vi "Navigation_no s curve may 2 encoders with mining.vi"() -> ()   [LabVIEW 2015]
uses:
  <vilib>/myRIO/Instrument Drivers/Onboard IO/PWM/typedefs/PWM Reference.ctl
  <vilib>/myRIO/Common/Instrument Driver Framework/Utilities/typedefs/myRIO Generic Hardware Reference.ctl
  <vilib>/myRIO/Common/Instrument Driver Framework/Utilities/typedefs/Hardware Version Enum.ctl
  <vilib>/myRIO/Common/Instrument Driver Framework/Utilities/typedefs/myRIO v1.0 Reference.ctl
  <vilib>/myRIO/Common/Instrument Driver Framework/Utilities/typedefs/Generic FPGA Reference.ctl
  <vilib>/myRIO/Common/Instrument Driver Framework/myRIO v1.0/PWM/typedefs/PWM Channels Enum.ctl
  <vilib>/myRIO/Instrument Drivers/Onboard IO/PWM/typedefs/PWM Configuration.ctl
  <vilib>/userdefined/High Color/nirio_resource_hc.ctl
  <vilib>/myRIO/Common/Instrument Driver Framework/myRIO v1.0/PWM/vis/myRIO v1.1 Open PWM.vi
  <vilib>/myRIO/Common/Instrument Driver Framework/Utilities/vis/Validate Channels.vi
  <vilib>/myRIO/Common/Instrument Driver Framework/myRIO v1.0/PWM/vis/myRIO v1.0 Reserve PWM.vi
  <vilib>/myRIO/Common/Instrument Driver Framework/myRIO v1.0/PWM/vis/myRIO v1.0 Build MUX Configuration PWM.vi
  <vilib>/myRIO/Common/Instrument Driver Framework/myRIO v1.0/Resource Manager/vis/myRIO v1.0 Reserve Channel List.vi
  <vilib>/myRIO/Common/Instrument Driver Framework/myRIO v1.0/Resource Manager/vis/myRIO v1.0 Create Configuration List.vi
  <vilib>/myRIO/Common/Instrument Driver Framework/myRIO v1.0/Resource Manager/vis/myRIO v1.0 Reserve Channel.vi
  <vilib>/myRIO/Common/Instrument Driver Framework/myRIO v1.0/Resource Manager/vis/myRIO v1.0 Unreserve Channel.vi
  <vilib>/myRIO/Common/Instrument Driver Framework/myRIO v1.0/Resource Manager/vis/myRIO v1.0 Build Mutex Name.vi
  <vilib>/FPGAPlugInAG/myRIO-1900/niLvFpga_Open_myRIO-1900.vi
  <vilib>/rvi/interface/common/dynamic/niFpgaDynamicAddResources.vi
  <vilib>/myRIO/Common/Instrument Driver Framework/Utilities/vis/FPGA Ref Manager.vi
  <vilib>/Utility/error.llb/Error Cluster From Error Code.vi
  <vilib>/myRIO/Common/Instrument Driver Framework/Utilities/vis/Ref Counter.vi
  <vilib>/rvi/errors/niLvFpgaAdjustHostInterfaceError.vi
  <vilib>/Utility/VariantDataType/GetNumericInfo.vi
  <vilib>/myRIO/Common/Instrument Driver Framework/myRIO v1.0/myRIO v1.1 Open.vi
  <vilib>/myRIO/Common/Instrument Driver Framework/Utilities/vis/IO Manager.vi
  <vilib>/myRIO/Common/Instrument Driver Framework/Utilities/vis/Configuration Manager.vi
  <vilib>/myRIO/Common/Instrument Driver Framework/myRIO v1.0/Resource Manager/vis/myRIO v1.0 Configure IO.vi
  <vilib>/myRIO/Common/Instrument Driver Framework/myRIO v1.0/myRIO v1.0 Close.vi
  <vilib>/myRIO/Common/Instrument Driver Framework/myRIO v1.0/PWM/vis/myRIO v1.0 Write PWM.vi
  <vilib>/addons/control/pid/pid.llb/PID (DBL).vi
  <vilib>/rvi/interface/nirviOpenFPGA/nirviOpenFPGA.xnode
  FPGA Bitfiles/NavigationProjec_FPGATarget2_FPGAMainNavigati_PWPHW8gwDxI.lvbitx
  <vilib>/rvi/interface/nirviReadWriteControl/nirviReadWriteControl.xnode
  <vilib>/myRIO/Instrument Drivers/Onboard IO/PWM/vis/myRIO PWM Open.xnode
  <vilib>/myRIO/Instrument Drivers/Onboard IO/PWM/PWM.lvlib
  <vilib>/myRIO/Instrument Drivers/Utilities/Utilities.lvlib
  NiFpgaLv.dll
  <vilib>/rvi/interface/Simulation/niFpgaSimulationCallBeginRW.vi
  <vilib>/addons/control/pid/NI_PID_pid.lvlib
panel:
  in  "Tab Control":enum32{"Page 1", "Page 2"}(tab)
  out "percent to goal":dbl
  out "x goal current":dbl=8.0
  out "big red button":i16
  out "y1ahead":dbl
  out "angle error":dbl
  out "y desired":dbl
  out "slope desired":dbl
  out "orientation theta desired":dbl
  out "current angle":dbl
  out "current y":dbl
  out "current x":dbl
  out "mining angle":dbl
  out "mining y":dbl
  out "mining x":dbl
  out "mining location":dbl=1.0
  out "distance to goal":dbl
  out "loc_y":dbl
  out "loc_x":dbl
  out "loc_theta":dbl
  in  "motor killswitch":bool=TRUE
  in  "set start position":bool
  in  "dumping complete":bool
  in  "digging complete?":bool
  in  "position good?":bool
  in  "state":dbl
  in  "x goal":dbl=8.0
  in  "Encoder Reset":bool
  out "scale":dbl=1.0
  out "reset x y 2":dbl
  out "stop motors":dbl
  out "encoder stop switch":dbl=1.0
  out "left wheels actual pwm":dbl
  out "right wheels actual pwm":dbl
  out "desired pwm right":dbl
  out "desired pwm left":dbl
  out "left setpoint":dbl
  out "right setpoint":dbl
  in  "PID Settings":enum32{"Right PID PWM", "Left PID PWM"}(tab)
  in  "output range right":cluster{"output high":dbl, "output low":dbl}={"output high"=0.13333, "output low"=-0.13333} {"output low" format="%.6f"; "output high" format="%.5f"}
  in  "PID gains right":T1={"proportional gain (Kc)"=0.002, "integral time (Ti, min)"=7e-07, "derivative time (Td, min)"=0.0} {"derivative time (Td, min)" format="%.8f"; "integral time (Ti, min)" format="%.8f"; "proportional gain (Kc)" format="%.8f"}
  out "dt out (s) right":dbl format="%.3f"
  out "PID feedback Right":dbl
  out "Elapsed Time (s) Right":dbl caption="Elapsed Time (s)"
  in  "pid reset right":bool
  in  "output range left":cluster{"output high":dbl, "output low":dbl}={"output high"=0.13333, "output low"=-0.13333} {"output low" format="%.6f"; "output high" format="%.5f"}
  in  "PID gains left":T1={"proportional gain (Kc)"=0.002, "integral time (Ti, min)"=7e-07, "derivative time (Td, min)"=0.0} {"derivative time (Td, min)" format="%.8f"; "integral time (Ti, min)" format="%.8f"; "proportional gain (Kc)" format="%.8f"}
  out "dt out (s) left":dbl format="%.3f"
  out "PID feedback Left":dbl
  out "Elapsed Time (s) Left":dbl caption="Elapsed Time (s)"
  in  "pid reset left":bool
  out "start angle":dbl=1.0
  out "start x":dbl=1.0
  out "start y":dbl
  in  "stuff that i dont want to mess with right now":T2(tab)
  out "RM Linear Velocity (rot/s)":dbl
  out "RR Rot Velocity (rot/s)":dbl
  out "LR Rot Velocity (rot/s)":dbl
  out "LM Rot Velocity (rot/s)":dbl
  out "LF Rot Velocity (rot/s)":dbl
  out "RF Linear Velocity (rot/s)":dbl
  out "Tick Count(mSec) 2":u32 caption="Tick Count(mSec)"
  out "y traveled 2":dbl
  out "x traveled 2":dbl
  out "y position 2":dbl
  out "x position 2":dbl
  out "y dot 2":dbl
  out "distance traveled 2":dbl
  out "psi dot 2":dbl
  out "x dot 2":dbl
  out ".not. x? 2":bool
  out ".not. x? 3":bool
  out "goal reached":bool=TRUE
  out "avg ENC.B":dbl
  out "avg ENC.A":dbl
  out "ENC.B_c.CNTR":i32
  out "ENC.B_b.CNTR":i32
  out "ENC.B_a.CNTR":i32
  out "ENC.A_c.CNTR":i32
  out "ENC.A_b.CNTR":i32
  out "ENC.A_a.CNTR":i32
  out "stage set point parameters":T3(tab)
  in  "x straight 1 end":dbl=2.0
  in  "ypstart straight 1":dbl
  in  "ystart":dbl=1.0
  in  "yend straight 1":dbl=2.0
  in  "ypend straight 1":dbl
  out "a":dbl
  out "b":dbl
  out "c":dbl
  out "d":dbl
  out "x turn end":dbl=7.0
  out "x straight 2 end":dbl=10.0
  in  "mining y 1":dbl=2.0
  in  "mining angle 1":dbl
  in  "mining x 1":dbl=-8.0
  in  "mining angle -1":dbl
  in  "mining y -1":dbl=4.0
  in  "mining x -1":dbl=-8.0
  out "left pwm":dbl(graph)
  out "right pwm":dbl(graph)
  out "SYS.SELECTA":u8 format="%08b"
  in  "R Min Linear Velocity (ft/s)":dbl=-2.0 format="%#_13g"
  in  "R Max Linear Velocity (ft/s)":dbl=2.0 format="%#_13g"
  in  "L Min Linear Velocity (ft/s)":dbl=-2.0 format="%#_13g"
  in  "L Max Linear Velocity (ft/s)":dbl=2.0 format="%#_13g"
  out "Current Rot Velocity (rot/s)":T4(graph)
  # "Position Information"
  # "move cases along"
  # "end state 0\ngo to state 1"
  # "end state 1\ngo to state 2"
  # "end state 2\ngo to state 3"
  # "end state 3\ngo to state 4"
  # "end state 4\ngo to state 0"
  # "same thing, redundant \nbut can be changed to \nsomething useful later"
  # "this must be true to \ninitialize the routine"
  # "go through the 3\n movement cases"
  # "go through the 3\n movement cases"
  # "Stop Flags \n1=go \n0=stop"
  # "PWM Setpoint"
  # "Initial condtions"
  # "Encoder Values"
  # "Motor Control Parameters"
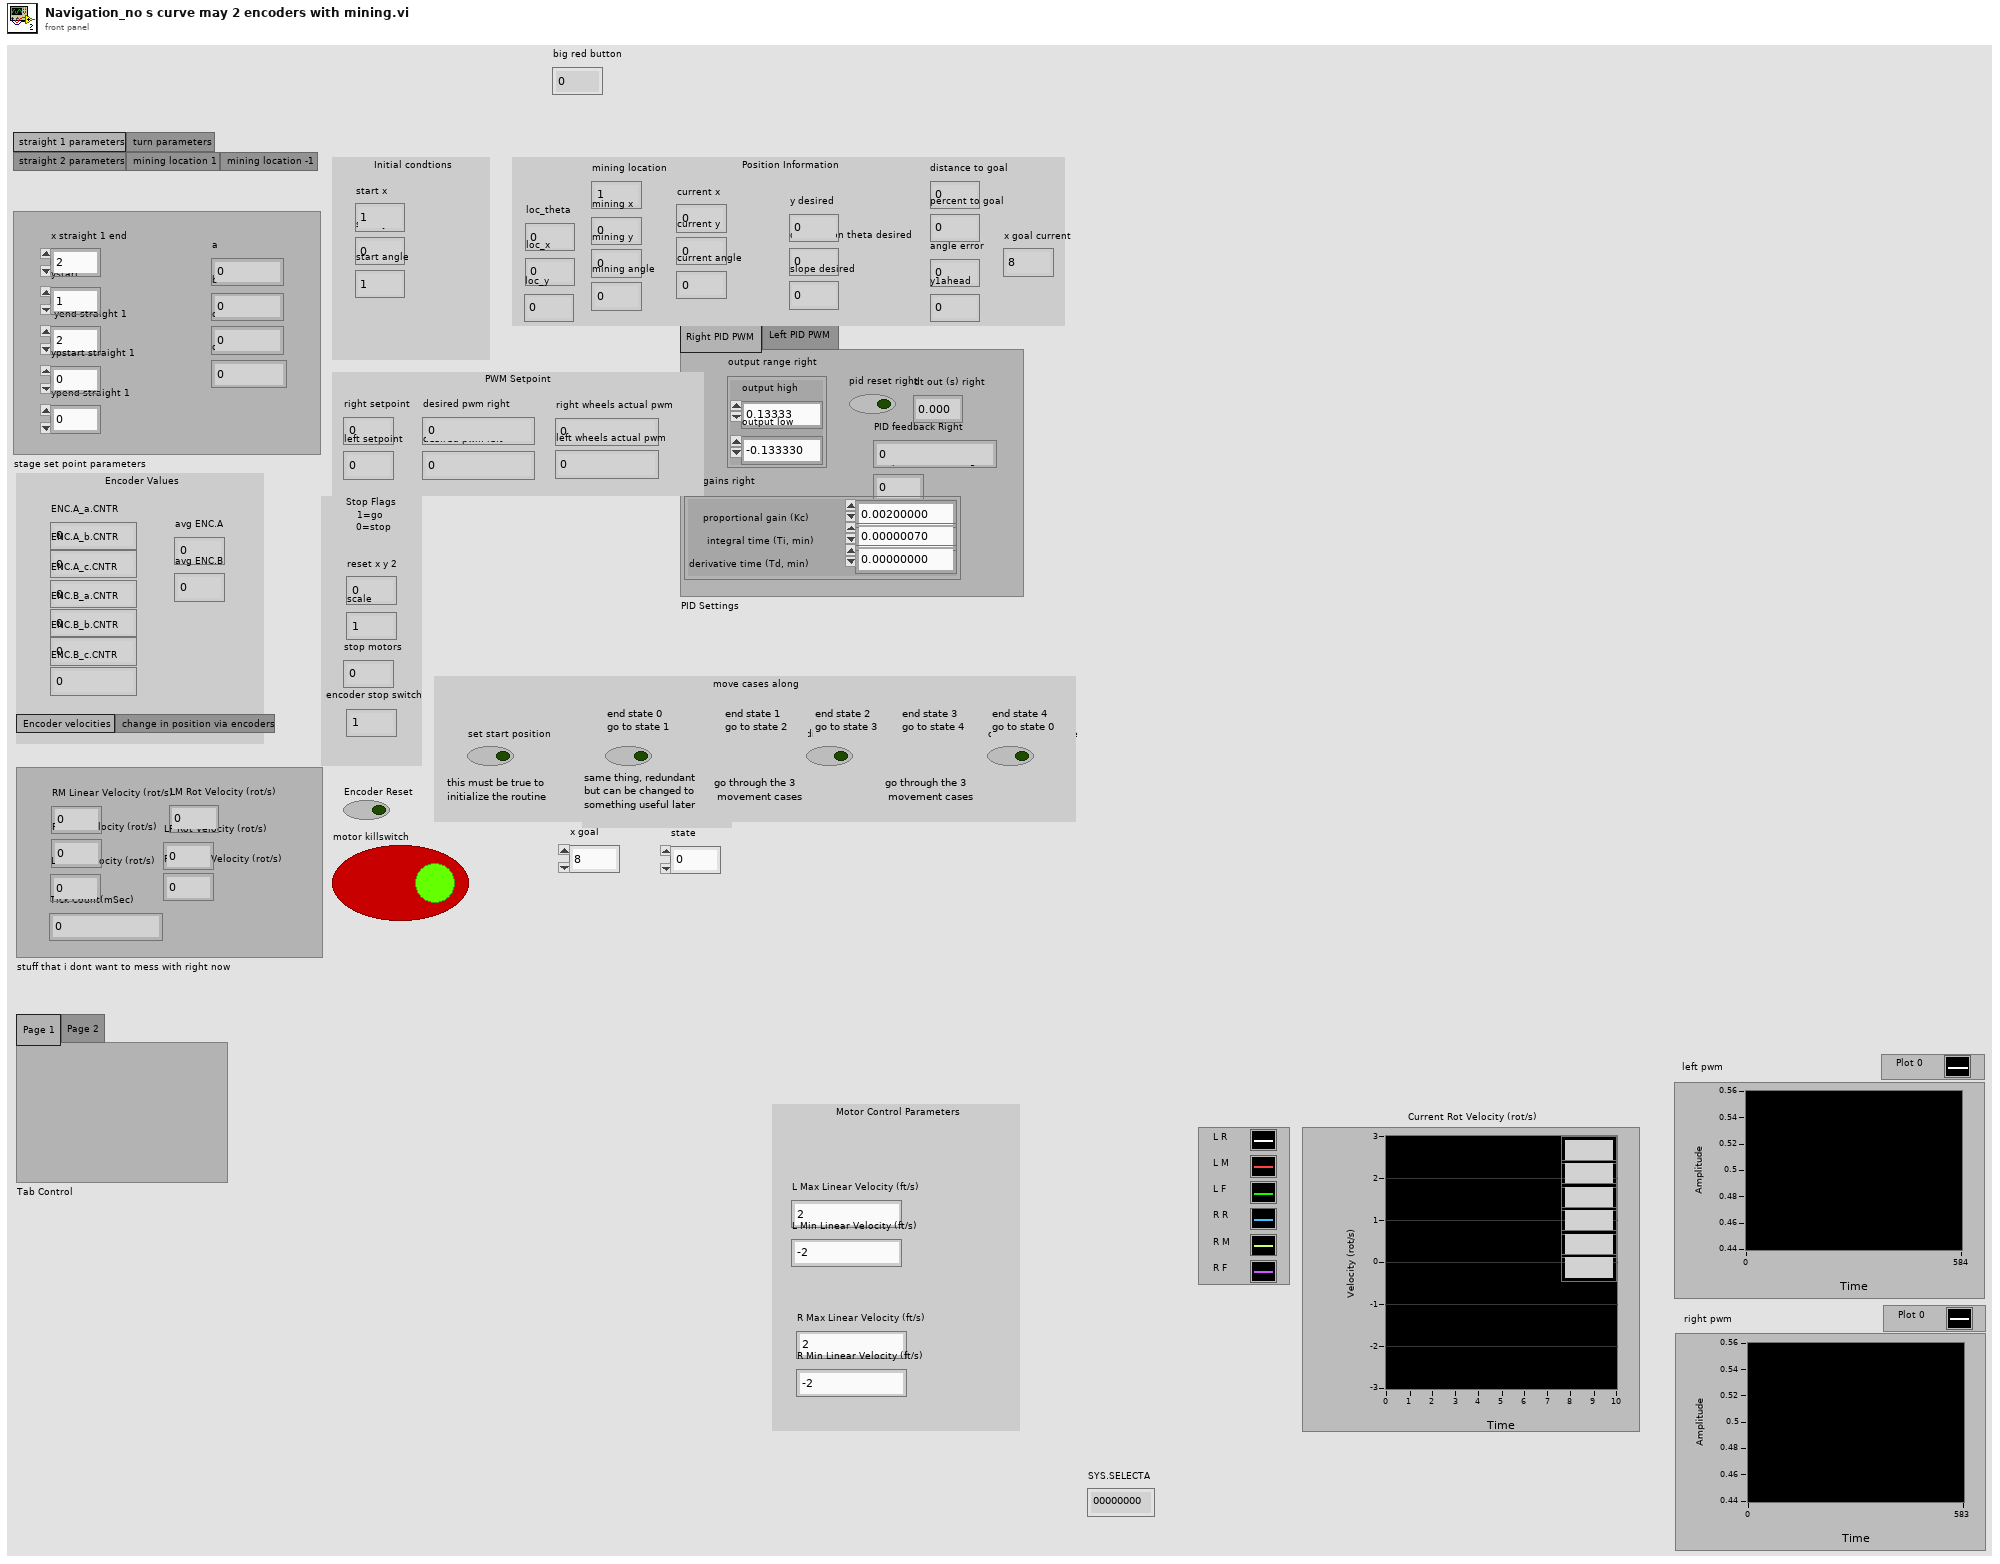
[diagram p1: front panel]
types:
  T1 = cluster{"proportional gain (Kc)":dbl, "integral time (Ti, min)":dbl, "derivative time (Td, min)":dbl}
  T2 = enum32{"Encoder velocities", "change in position via encoders"}
  T3 = enum32{"straight 1 parameters", "turn parameters", "straight 2 parameters", "mining location 1", "mining location -1"}
  T4 = cluster{"Rotational Velocity (RPS)":dbl, "Rotational Velocity (RPS)":dbl, "Rotational Velocity (RPS)":dbl, "Rotational Velocity (RPS)":dbl, "Rotational Velocity (RPS)":dbl, "Rotational Velocity (RPS)":dbl}
  T5 = typedef "nirio_resource_hc.ctl" = tag
  T6 = typedef "Hardware Version Enum.ctl" = enum16{"Unknown", "myRIO-1900", "myRIO-1950", "roboRIO"}
  T7 = typedef "PWM.lvlib/PWM Reference.ctl" = cluster{"myRIO Reference":T8, "PWM Channels Enum":T11, "PWM Configuration":T12}
  T8 = typedef "myRIO Generic Hardware Reference.ctl" = cluster{"myRIO Model":T6, "myRIO Hardware Reference":T9}
  T9 = typedef "myRIO v1.0 Reference.ctl" = cluster{"Generic FPGA Reference":T10, "Allow multiple opens":bool}
  T10 = typedef "Generic FPGA Reference.ctl" = refnum<k20>
  T11 = typedef "PWM Channels Enum.ctl" = enum16{"Not Connected", "C/PWM0", "C/PWM1", "A/PWM0", "A/PWM1", "A/PWM2", "B/PWM0", "B/PWM1", "B/PWM2", "PWM/PWM0", "PWM/PWM1", "PWM/PWM2", "PWM/PWM3", "PWM/PWM4", "PWM/PWM5", "PWM/PWM6", "PWM/PWM7", "PWM/PWM8", "PWM/PWM9"}
  T12 = typedef "PWM.lvlib/PWM Configuration.ctl" = cluster{"Frequency":dbl, "Duty Cycle":dbl}
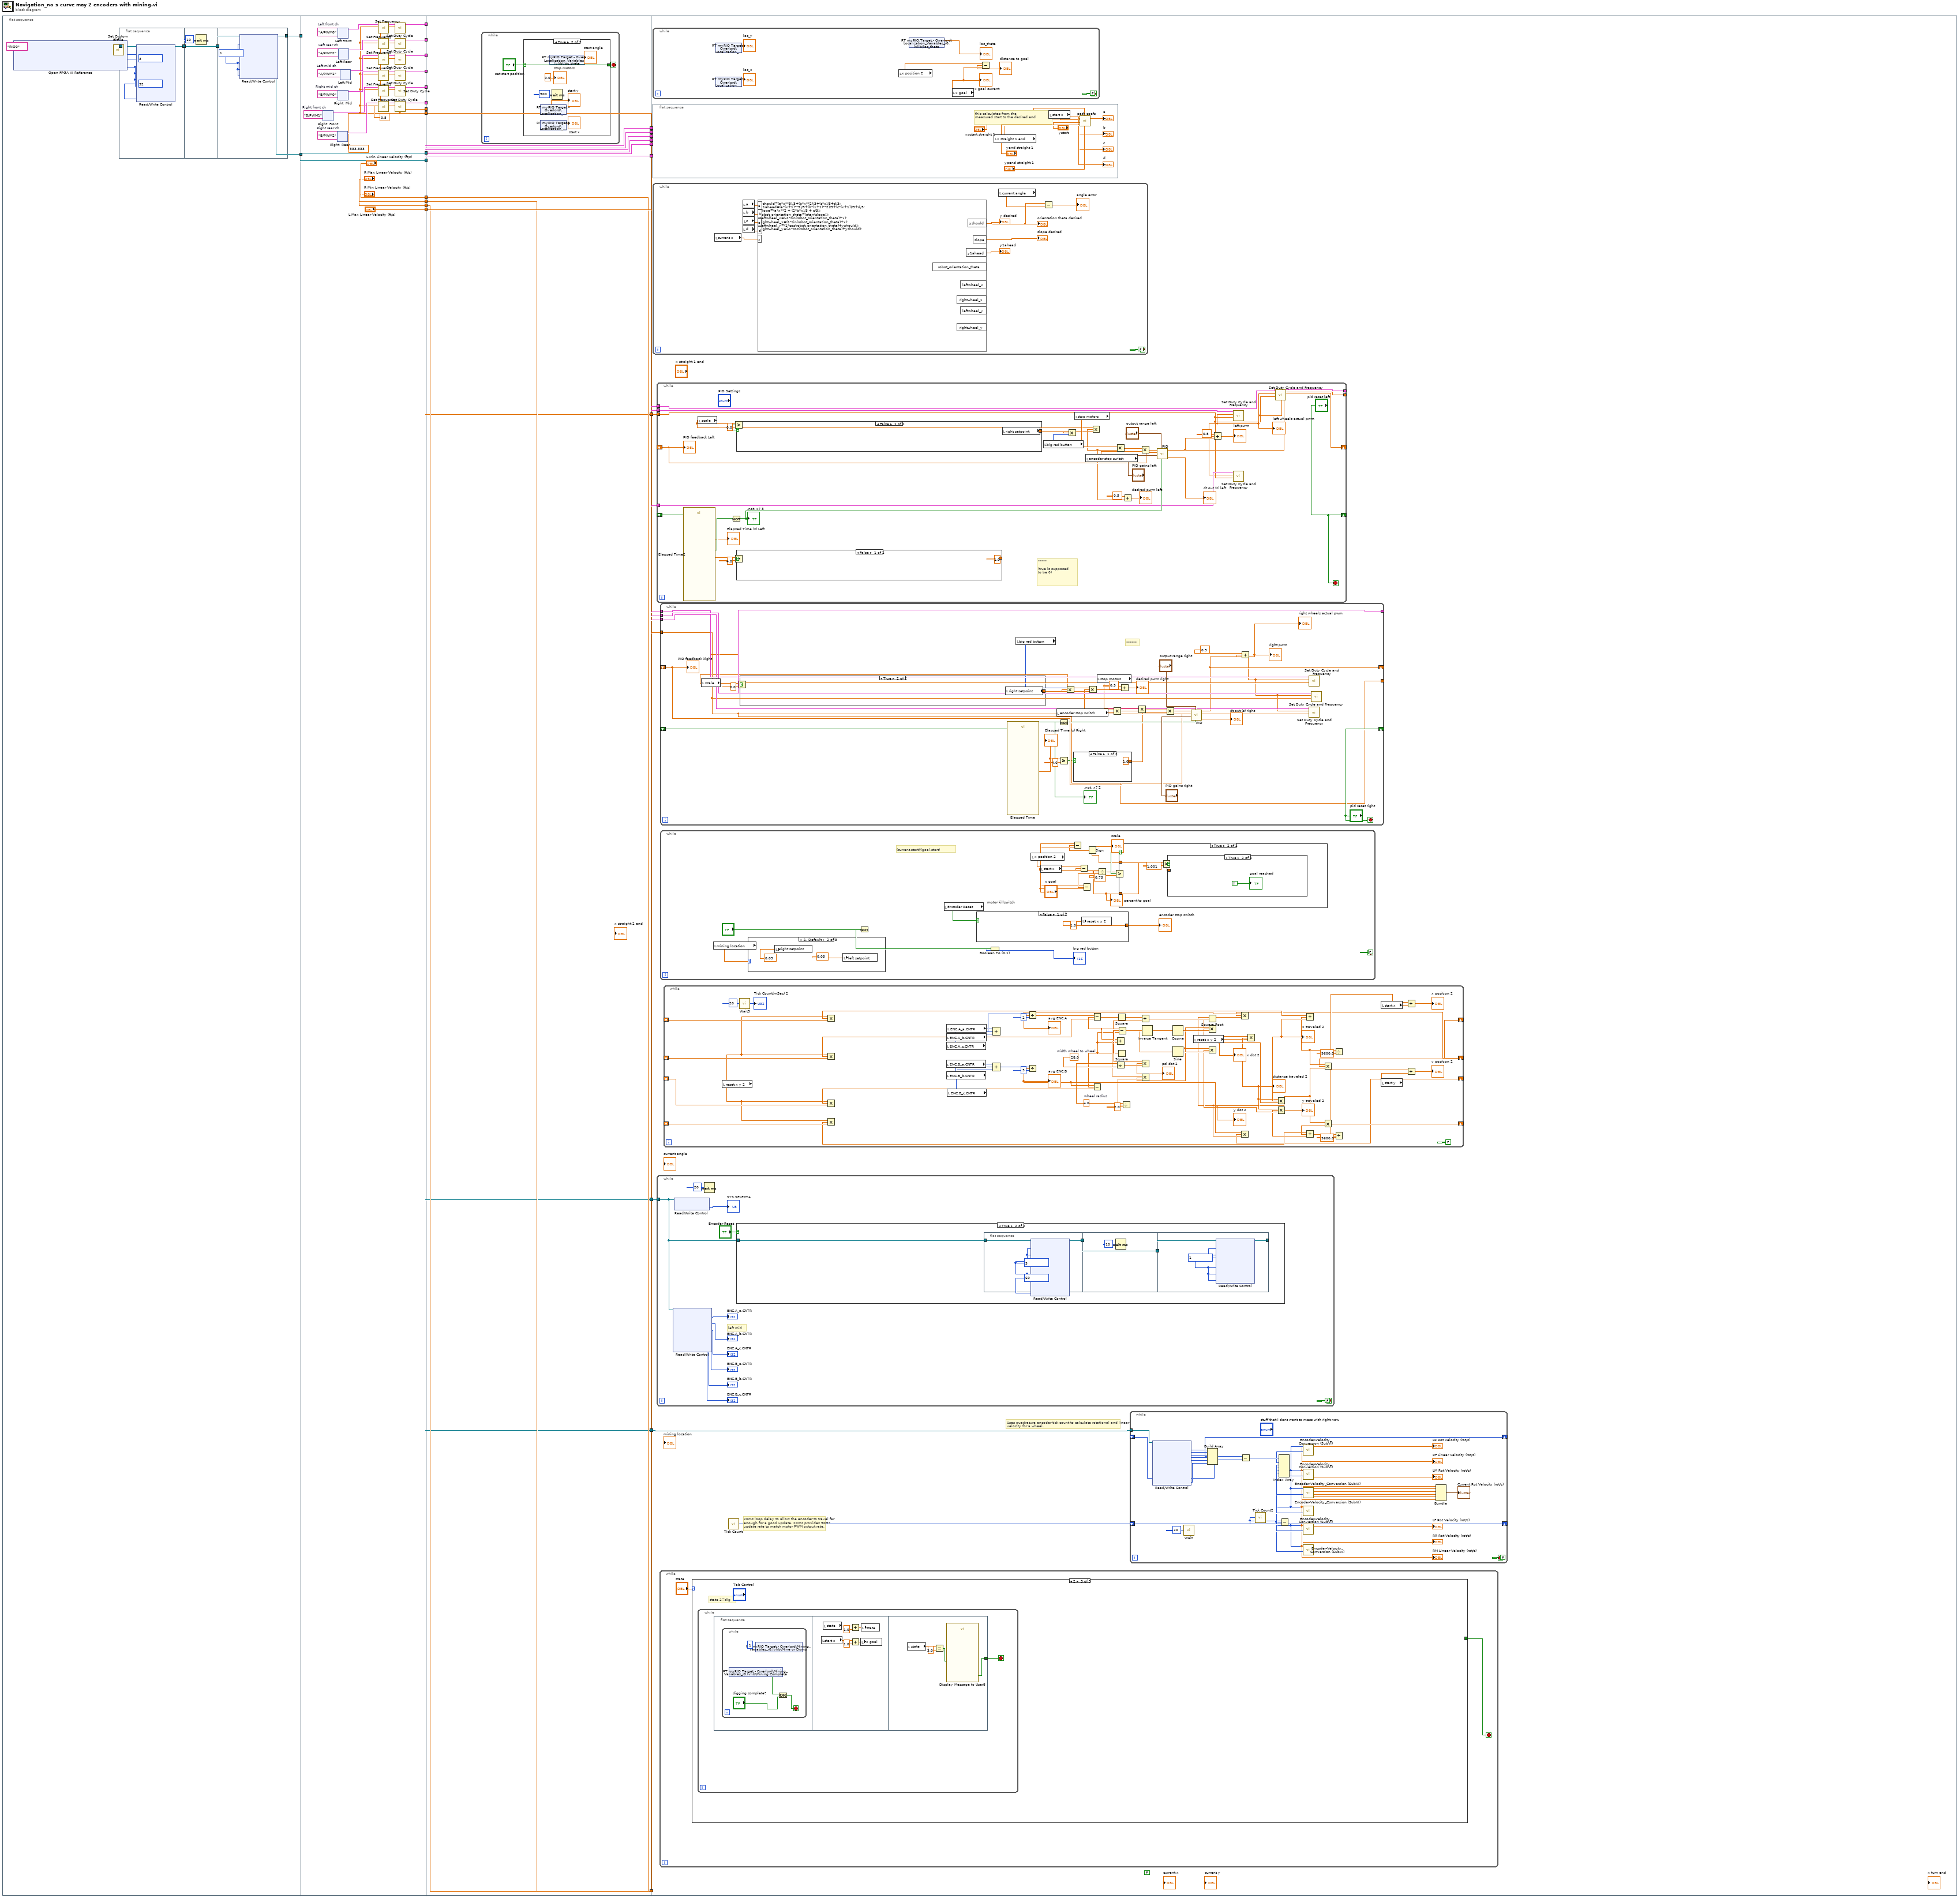
[diagram p0: block diagram]
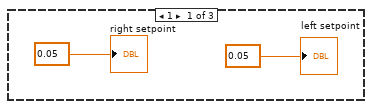
[diagram p3: hidden frame]
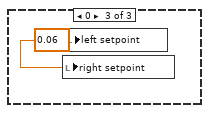
[diagram p4: hidden frame]
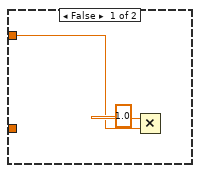
[diagram p5: hidden frame]
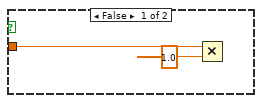
[diagram p6: hidden frame]
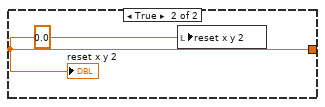
[diagram p7: hidden frame]
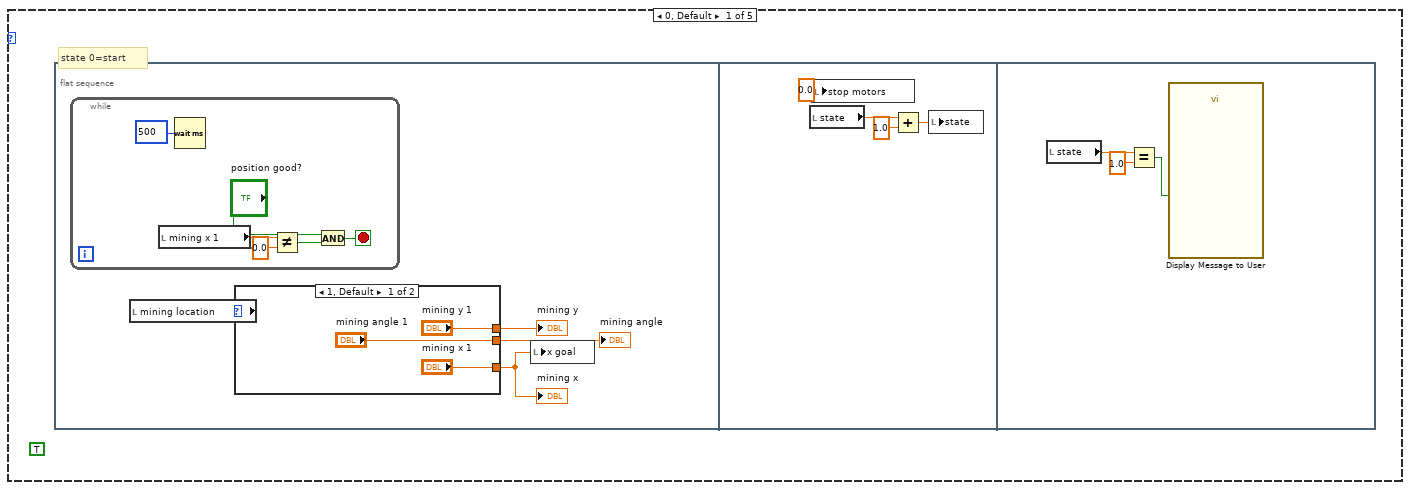
[diagram p8: hidden frame]
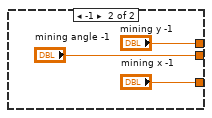
[diagram p9: hidden frame]
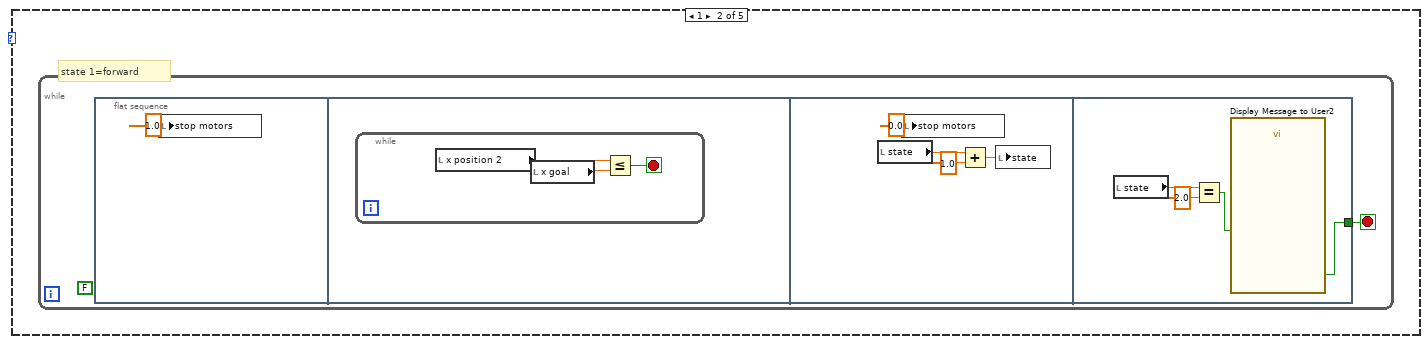
[diagram p10: hidden frame]
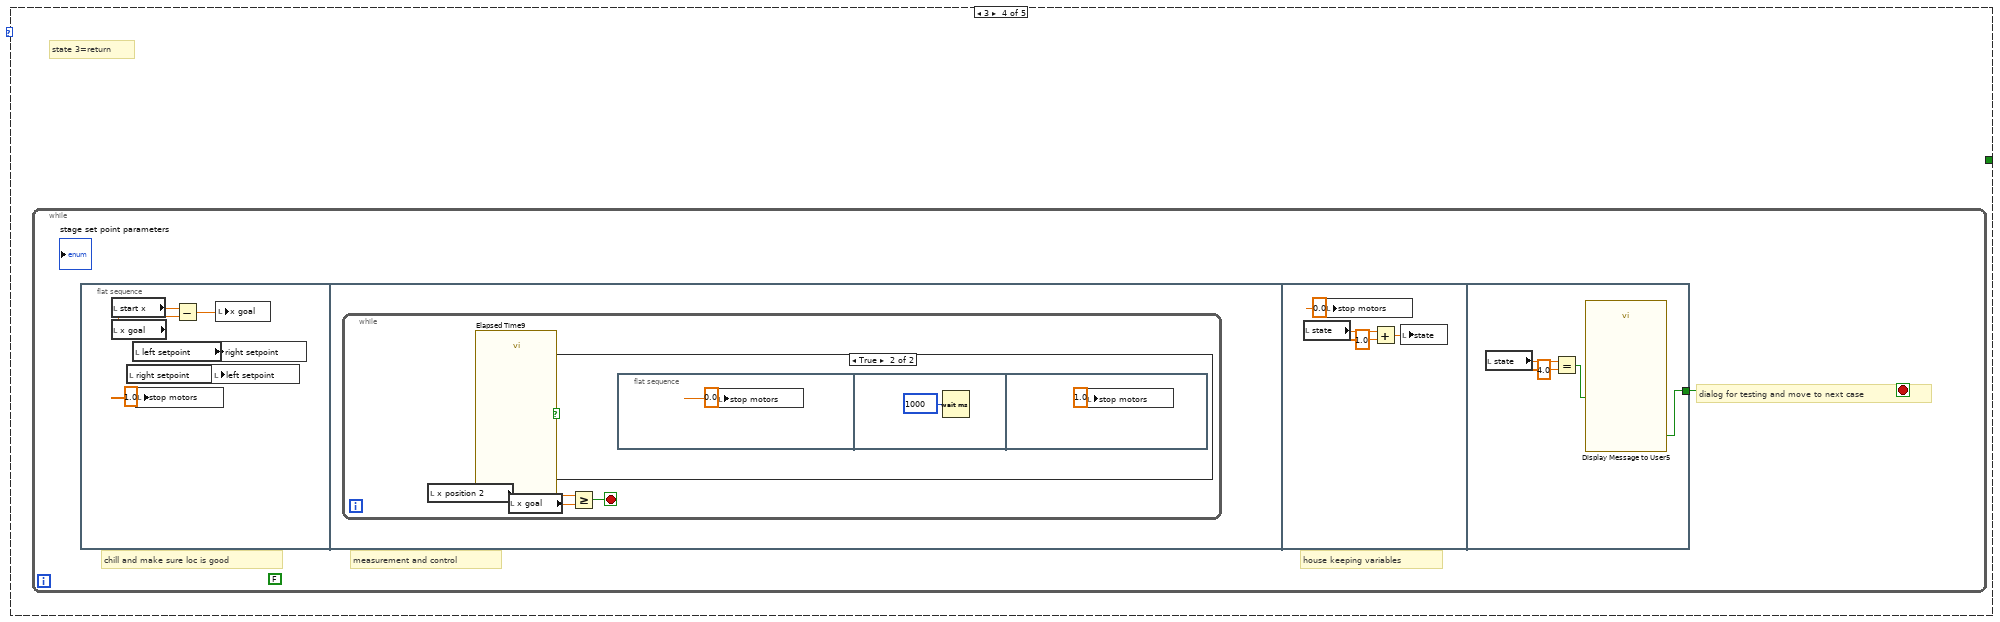
[diagram p11: hidden frame]
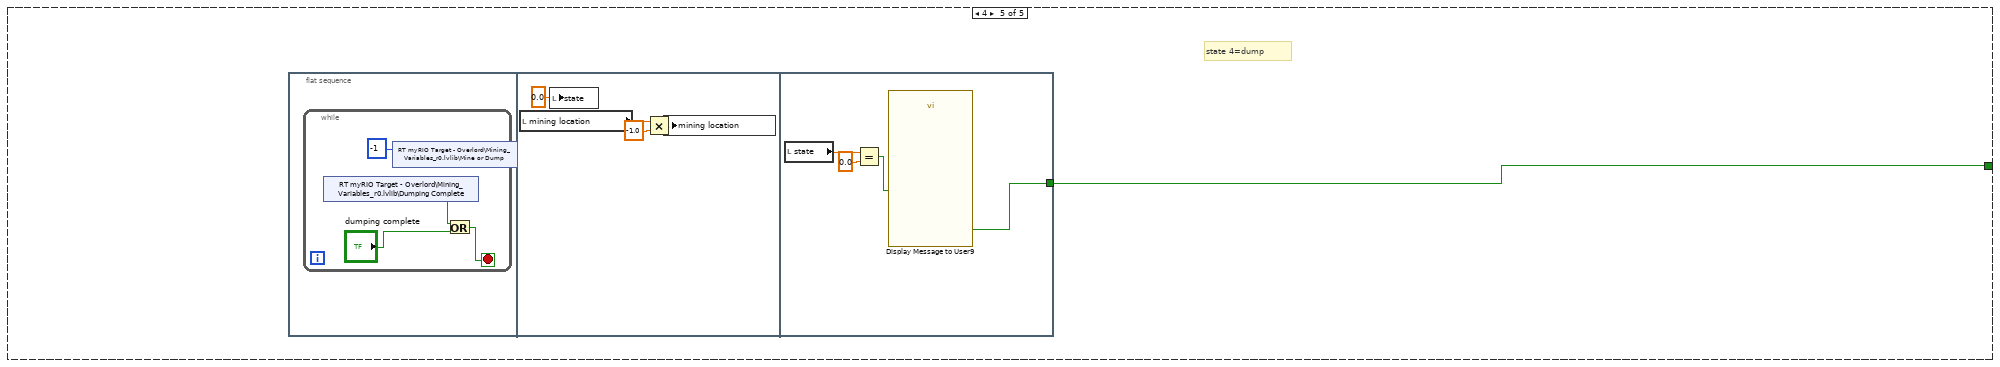
[diagram p13: hidden frame]
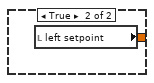
[diagram p14: hidden frame]
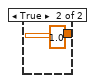
[diagram p15: hidden frame]
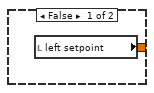
[diagram p16: hidden frame]
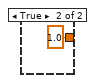
[diagram p17: hidden frame]
diagram:
  n1 = flat-sequence {
    tunnel: [w33] -> w30
    tunnel: [w33] -> w29
    tunnel: [w46] -> w28
    tunnel: [w61] -> w26
    tunnel: [w57] -> w24
    tunnel: [w56] -> w22
    tunnel: [w55] -> w20
    tunnel: [w54] -> w18
    tunnel: [w53] -> w16
    tunnel: ["L Max Linear Velocity (ft/s)"] -> w14
    tunnel: ["L Min Linear Velocity (ft/s)"] -> w12
    tunnel: ["R Max Linear Velocity (ft/s)"] -> w10
    tunnel: ["R Min Linear Velocity (ft/s)"] -> w8
    tunnel: [w48] -> w6
    tunnel: w30 -> [w47]
    tunnel: [w47] -> w4
    tunnel: w29 -> [w48]
    tunnel: [w46] -> w2
    tunnel: w28 -> [w187]
    tunnel: [w187] -> w27
    tunnel: w26 -> [w186]
    tunnel: [w186] -> w25
    tunnel: w24 -> [w185]
    tunnel: [w185] -> w23
    tunnel: w22 -> [w184]
    tunnel: [w184] -> w21
    tunnel: w20 -> [w183]
    tunnel: [w183] -> w19
    tunnel: w18 -> [w182]
    tunnel: [w182] -> w17
    tunnel: w16 -> [w181]
    tunnel: [w181] -> w15
    tunnel: w14 -> [w180]
    tunnel: [w180] -> w13
    tunnel: w12 -> [w179]
    tunnel: [w179] -> w11
    tunnel: w10 -> [w178]
    tunnel: [w178] -> w9
    tunnel: w8 -> [w177]
    tunnel: [w177] -> w7
    tunnel: w6 -> [w176]
    tunnel: [w176] -> w5
    tunnel: w4 -> [w175]
    tunnel: [w175] -> w3
    tunnel: w2 -> [w174]
    tunnel: [w174] -> w1
    tunnel: w27 -> [_]
    tunnel: w25 -> [w196]
    tunnel: w23 -> [w202]
    tunnel: w21 -> [w199]
    tunnel: w19 -> [w198]
    tunnel: w17 -> [w197]
    tunnel: w15 -> [w201]
    tunnel: w13 -> [_]
    tunnel: w11 -> [_]
    tunnel: w9 -> [_]
    tunnel: w7 -> [_]
    tunnel: w5 -> [w204]
    tunnel: w3 -> [w203]
    tunnel: w1 -> [w200]
    frame #0 {
      n2 = xnode "Open FPGA VI Reference"("resource name"=tag "RIO0") -> ("FPGA VI Reference Out"=w32:refnum<k20>)  [unwired: 1 in, 1 out]
      n3 = call <vilib>:"Set Custom Bitfile.vi"("Custom FPGA Reference In"=w32) -> ("Custom FPGA Reference Out"=w34:refnum<k20>)  [unwired: 9 in, 1 out]
      n4 = flat-sequence {
        tunnel: w34 -> [w39]
        tunnel: [w37] -> w36
        tunnel: w36 -> [w41]
        tunnel: [w41] -> w35
        tunnel: w35 -> [w44]
        tunnel: [w43] -> w33
        frame #0 {
          w38 = u8 32 ("SYS.SELECTA")
          w40 = u8 3 ("ENC.B_c.CNFG")
          n5 = xnode "Read/Write Control"("FPGA VI Reference In"=w39, "ENC.A_a.CNFG"=w40, "ENC.A_b.CNFG"=w40, "ENC.A_c.CNFG"=w40, "ENC.B_a.CNFG"=w40, "ENC.B_b.CNFG"=w40, "ENC.B_c.CNFG"=w40, "SYS.SELECTA"=w38, "SYS.SELECTB"=w38) -> ("FPGA VI Reference Out"=w37:refnum<k20>)  [unwired: 1 in, 1 out]
        }
        frame #1 {
          n6 = Wait (ms)(milliseconds to wait=u32 10) -> ()  [unwired: 1 out]
        }
        frame #2 {
          w45 = u8 1 ("ENC.B_c.CNFG")
          n7 = xnode "Read/Write Control"("FPGA VI Reference In"=w44, "ENC.A_a.CNFG"=w45, "ENC.A_b.CNFG"=w45, "ENC.A_c.CNFG"=w45, "ENC.B_a.CNFG"=w45, "ENC.B_b.CNFG"=w45, "ENC.B_c.CNFG"=w45) -> ("FPGA VI Reference Out"=w43:refnum<k20>)  [unwired: 1 in, 1 out]
        }
      }
    }
    frame #1 {
      w58 = 0.5 ("Duty Cycle")
      w46 = 333.333 ("Frequency [Hz]")
      w72 = tag "B/PWM2"  # Right rear ch
      w73 = tag "B/PWM0"  # Right mid ch
      w74 = tag "B/PWM1"  # Right front ch
      w75 = tag "A/PWM2"  # Left rear ch
      w76 = tag "A/PWM1"  # Left mid ch
      w77 = tag "A/PWM0"  # Left front ch
      n8 = xnode "Right  Front"("Channel Name"=w74) -> ("PWM Ref Out"=w68:T7)  [unwired: 2 in, 1 out]
      n9 = xnode "Right  Rear"("Channel Name"=w72) -> ("PWM Ref Out"=w66:T7)  [unwired: 2 in, 1 out]
      n10 = xnode "Left Front"("Channel Name"=w77) -> ("PWM Ref Out"=w71:T7)  [unwired: 2 in, 1 out]
      n11 = xnode "Right  Mid"("Channel Name"=w73) -> ("PWM Ref Out"=w67:T7)  [unwired: 2 in, 1 out]
      n12 = xnode "Left Rear"("Channel Name"=w75) -> ("PWM Ref Out"=w69:T7)  [unwired: 2 in, 1 out]
      n13 = xnode "Left Mid"("Channel Name"=w76) -> ("PWM Ref Out"=w70:T7)  [unwired: 2 in, 1 out]
      n14 = call <vilib>:"Set Frequency.vi"("Frequency [Hz]"=w46, "PWM Ref In"=w71) -> ("PWM Ref Out"=w65:T7)  [unwired: 7 in, 1 out]
      n15 = call <vilib>:"Set Frequency.vi"("Frequency [Hz]"=w46, "PWM Ref In"=w69) -> ("PWM Ref Out"=w60:T7)  [unwired: 7 in, 1 out]
      n16 = call <vilib>:"Set Frequency.vi"("Frequency [Hz]"=w46, "PWM Ref In"=w70) -> ("PWM Ref Out"=w59:T7)  [unwired: 7 in, 1 out]
      n17 = call <vilib>:"Set Frequency.vi"("Frequency [Hz]"=w46, "PWM Ref In"=w67) -> ("PWM Ref Out"=w63:T7)  [unwired: 7 in, 1 out]
      n18 = call <vilib>:"Set Frequency.vi"("Frequency [Hz]"=w46, "PWM Ref In"=w68) -> ("PWM Ref Out"=w62:T7)  [unwired: 7 in, 1 out]
      n19 = call <vilib>:"Set Frequency.vi"("Frequency [Hz]"=w46, "PWM Ref In"=w66) -> ("PWM Ref Out"=w64:T7)  [unwired: 7 in, 1 out]
      n20 = call <vilib>:"Set Duty Cycle.vi"("Duty Cycle"=w58, "PWM Ref In"=w65) -> ("PWM Ref Out"=w53:T7)  [unwired: 7 in, 1 out]
      n21 = call <vilib>:"Set Duty Cycle.vi"("Duty Cycle"=w58, "PWM Ref In"=w60) -> ("PWM Ref Out"=w61:T7)  [unwired: 7 in, 1 out]
      n22 = call <vilib>:"Set Duty Cycle.vi"("Duty Cycle"=w58, "PWM Ref In"=w59) -> ("PWM Ref Out"=w54:T7)  [unwired: 7 in, 1 out]
      n23 = call <vilib>:"Set Duty Cycle.vi"("Duty Cycle"=w58, "PWM Ref In"=w63) -> ("PWM Ref Out"=w56:T7)  [unwired: 7 in, 1 out]
      n24 = call <vilib>:"Set Duty Cycle.vi"("Duty Cycle"=w58, "PWM Ref In"=w62) -> ("PWM Ref Out"=w57:T7)  [unwired: 7 in, 1 out]
      n25 = call <vilib>:"Set Duty Cycle.vi"("Duty Cycle"=w58, "PWM Ref In"=w64) -> ("PWM Ref Out"=w55:T7)  [unwired: 7 in, 1 out]
    }
    frame #2 {
      n26 = while {
        stop <- w188 stop-if-true
        n27 = case shown="True" "set start position" {
          selector: "set start position" -> [_ w195]
          tunnel: [_ w195] -> w188
          frame False {
          }
          frame True {
            n28 = shared-variable "RT myRIO Target - Overlord\\Localization_Variables_r0.lvlib\\loc_y"() -> (→"start y":dbl)  [unwired: 1 in, 1 out]
            n29 = shared-variable "RT myRIO Target - Overlord\\Localization_Variables_r0.lvlib\\loc_x"() -> (→"start x":dbl)  [unwired: 1 in, 1 out]
            n30 = shared-variable "RT myRIO Target - Overlord\\Localization_Variables_r0.lvlib\\loc_theta"() -> (→"start angle":dbl)  [unwired: 1 in, 1 out]
            n31 = Wait (ms)(milliseconds to wait=u32 500) -> ()  [unwired: 1 out]
            "stop motors" <- 0.0 ("stop motors")
          }
        }
      }
    }
    frame #3 {
      (unwired) FALSE
      # "Uses quadrature encoder tick count to calculate rotational and linear velocity for a wheel."
      # "20ms loop delay to allow the encoder to travel far enough for a good update. 20ms provides 50Hz update rate to match motor PWM output rate."
      n32 = while {
        stop <- FALSE stop-if-true
        n33 = shared-variable "RT myRIO Target - Overlord\\Localization_Variables_r0.lvlib\\loc_y"() -> (→"loc_y":dbl)  [unwired: 1 in, 1 out]
        n34 = shared-variable "RT myRIO Target - Overlord\\Localization_Variables_r0.lvlib\\loc_x"() -> (→"loc_x":dbl)  [unwired: 1 in, 1 out]
        n35 = local read "x position 2"() -> (w349:dbl)
        n36 = shared-variable "RT myRIO Target - Overlord\\Localization_Variables_r0.lvlib\\loc_theta"() -> (→"loc_theta":dbl)  [unwired: 1 in, 1 out]
        n37 = local read "x goal"() -> (w352:dbl)
        "x goal current" <- w352
        n38 = Subtract(x=w349, y=w352) -> (x-y=→"distance to goal":dbl)
      }
      n39 = flat-sequence {
        frame #0 {
          # "this calculates from the \nmeasured start to the desired end"
          n40 = local read "x straight 1 end"() -> (w251:dbl)
          n41 = local read "start x"() -> (w252:dbl)
          n42 = call "path coefs.vi"("ypend"="ypend straight 1", "ypstart"="ypstart straight 1", "yend"="yend straight 1", "ystart"="ystart", "xend"=w251, "xstart"=w252) -> ("d"=→"d":dbl, "c"=→"c":dbl, "b"=→"b":dbl, "a"=→"a":dbl)  [unwired: 2 in]
        }
      }
      n43 = while {
        stop <- FALSE stop-if-true
        n44 = local read "current x"() -> (w245:dbl)
        n45 = local read "a"() -> (w249:dbl)
        n46 = local read "b"() -> (w248:dbl)
        n47 = local read "d"() -> (w246:dbl)
        n48 = local read "c"() -> (w247:dbl)
        n49 = formula code="yshould=(a*x**3)/3+(b*x**2)/3+(c*x)/3+d/3;\ny1ahead=(a*(x+1)**3)/3+(b*(x+1)**2)/3+(c*(x+1))/3+d/3;\nslope=(a*x**2 + (2*b*x)/3 + c/3);\nrobot_orientation_theta=(atan(slope));\nleftwheel_x=(-1*sin(robot_orientation_theta)+x);\nrightwheel_x=(1*sin(robot_orientation_theta)+x);\nleftwheel_y=(1*cos(robot_orientation_theta)+yshould);\nrightwheel_y=(-1*cos(robot_orientation_theta)+yshould);"("a"=w249, "b"=w248, "c"=w247, "d"=w246, "x"=w245) -> ("yshould"=→"y desired":dbl, "slope"=→"slope desired":dbl, "robot_orientation_theta"=w242:dbl, "y1ahead"=→"y1ahead":dbl)  [unwired: 4 out]
        "orientation theta desired" <- w242
        n50 = local read "current angle"() -> (w241:dbl)
        n51 = Subtract(x=w242, y=w241) -> (x-y=→"angle error":dbl)
      }
      n52 = while {
        tunnel: w201 -> [w386]
        tunnel: [w387] -> _
        tunnel: w200 -> [w374]
        shift-right: [w373] -> _
        shift-left: _ -> [w382]
        shift-right: ["pid reset left"] -> _
        shift-left: _ -> [w368]
        tunnel: [w374] -> _
        tunnel: w197 -> [w376]
        tunnel: w196 -> [w375]
        stop <- "pid reset left" stop-if-true
        # "*****\n\n(true is supposed\nto be 0)"
        n53 = call "Elapsed Time2"("Reset"=w368) -> ("Elapsed Time (s)"=w367:dbl, "Time has Elapsed"=w369:bool)  [unwired: 11 in, 6 out]
        "Elapsed Time (s) Left" <- w367
        n54 = local read "scale"() -> (w359:dbl)
        n55 = Not(x=w369) -> (.not. x?=w381:bool)
        ".not. x? 3" <- w381
        n56 = Greater?(x=w359, y=0.0) -> (0:w362:bool)
        n57 = Greater Or Equal?(x=w367, y=4.0) -> (x >= y?=w365:bool)
        n58 = case shown="False" w362 {
          tunnel: [w388 w389] -> w372
          frame False {
            n59 = local read "right setpoint"() -> (w388:dbl)
          }
          frame True {
            n60 = local read "left setpoint"() -> (w389:dbl)
          }
        }
        n61 = case shown="False" w365 {
          tunnel: [1.0 1.0] -> _
          frame False {
          }
          frame True {
          }
        }
        n62 = local read "big red button"() -> (w356:i16)
        n63 = Multiply(x=w372, y=w356) -> (x*y=w357:dbl)
        n64 = local read "stop motors"() -> (w377:dbl)
        n65 = local read "encoder stop switch"() -> (w370:dbl)
        n66 = Multiply(x=w359, y=w357) -> (x*y=w360:dbl)
        n67 = Multiply(x=w377, y=w360) -> (x*y=w371:dbl)
        n68 = Add(x=0.5, y=w360) -> (x+y=→"desired pwm left":dbl)
        n69 = Multiply(x=w371, y=w370) -> (x*y=w358:dbl)
        n70 = call-poly <vilib>:"PID.vi"("reinitialize? (F)"=w381, "output range"="output range left", "PID gains"="PID gains left", "process variable"=w382, "setpoint"=w358) -> ("dt out (s)"=→"dt out (s) left":dbl, "output"=w373:dbl)  [unwired: 5 in]
        n71 = Add(x=0.5, y=w373) -> (x+y=w363:dbl)
        "left wheels actual pwm" <- w363
        "left pwm" <- w363
        n72 = call <vilib>:"Set Duty Cycle and Frequency.vi"("Frequency [Hz]"=w374, "Duty Cycle"=w363, "PWM Ref In"=w375) -> ()  [unwired: 6 in, 2 out]
        n73 = call <vilib>:"Set Duty Cycle and Frequency.vi"("Frequency [Hz]"=w374, "Duty Cycle"=w363, "PWM Ref In"=w376) -> ()  [unwired: 6 in, 2 out]
        n74 = call <vilib>:"Set Duty Cycle and Frequency.vi"("Frequency [Hz]"=w374, "Duty Cycle"=w363, "PWM Ref In"=w386) -> ("PWM Ref Out"=w387:T7)  [unwired: 6 in, 1 out]
        "PID feedback Left" <- w382
      }
      n75 = while {
        tunnel: w204 -> [w492]
        stop <- FALSE stop-if-true
        # "left mid"
        n76 = xnode "Read/Write Control"("FPGA VI Reference In"=w492) -> ("ENC.A_a.CNTR"=→"ENC.A_a.CNTR":u32, "ENC.A_b.CNTR"=→"ENC.A_b.CNTR":u32, "ENC.A_c.CNTR"=→"ENC.A_c.CNTR":u32, "ENC.B_a.CNTR"=→"ENC.B_a.CNTR":u32, "ENC.B_b.CNTR"=→"ENC.B_b.CNTR":u32, "ENC.B_c.CNTR"=→"ENC.B_c.CNTR":u32)  [unwired: 1 in, 2 out]
        n77 = xnode "Read/Write Control"("FPGA VI Reference In"=w492) -> ("SYS.SELECTA"=→"SYS.SELECTA":u8)  [unwired: 1 in, 2 out]
        n78 = Wait (ms)(milliseconds to wait=u32 20) -> ()  [unwired: 1 out]
        n79 = case shown="True" "Encoder Reset" {
          tunnel: w492 -> [_ w503]
          frame False {
          }
          frame True {
            n80 = flat-sequence {
              tunnel: w503 -> [w508]
              tunnel: [w506] -> w505
              tunnel: w505 -> [w510]
              tunnel: [w510] -> w504
              tunnel: w504 -> [w513]
              tunnel: [w512] -> _
              frame #0 {
                w507 = u8 60 ("SYS.SELECTA")
                w509 = u8 3 ("ENC.B_c.CNFG")
                n81 = xnode "Read/Write Control"("FPGA VI Reference In"=w508, "ENC.A_a.CNFG"=w509, "ENC.A_b.CNFG"=w509, "ENC.A_c.CNFG"=w509, "ENC.B_a.CNFG"=w509, "ENC.B_b.CNFG"=w509, "ENC.B_c.CNFG"=w509, "SYS.SELECTA"=w507, "SYS.SELECTB"=w507) -> ("FPGA VI Reference Out"=w506:refnum<k20>)  [unwired: 1 in, 1 out]
              }
              frame #1 {
                n82 = Wait (ms)(milliseconds to wait=u32 10) -> ()  [unwired: 1 out]
              }
              frame #2 {
                w514 = u8 1 ("ENC.B_c.CNFG")
                n83 = xnode "Read/Write Control"("FPGA VI Reference In"=w513, "ENC.A_a.CNFG"=w514, "ENC.A_b.CNFG"=w514, "ENC.A_c.CNFG"=w514, "ENC.B_a.CNFG"=w514, "ENC.B_b.CNFG"=w514, "ENC.B_c.CNFG"=w514) -> ("FPGA VI Reference Out"=w512:refnum<k20>)  [unwired: 1 in, 1 out]
              }
            }
          }
        }
      }
      n84 = while {
        stop <- w262 stop-if-true
        n85 = case shown="2" "state" {
          tunnel: [_ _ _ _ w336] -> w262
          frame 0, Default {
            (unwired) TRUE
            # "state 0=start"
            n86 = flat-sequence {
              frame #0 {
                n87 = while {
                  stop <- w273 stop-if-true
                  n88 = local read "mining x 1"() -> (w278:dbl)
                  n89 = Wait (ms)(milliseconds to wait=u32 500) -> ()  [unwired: 1 out]
                  n90 = Not Equal?(x=w278, y=0.0) -> (x != y?=w274:bool)
                  n91 = And(x="position good?", y=w274) -> (x .and. y?=w273:bool)
                }
                n92 = local read "mining location"() -> (w266:dbl)
                n93 = case shown="1, Default" w266 {
                  tunnel: ["mining x 1" "mining x -1"] -> w263
                  tunnel: ["mining y 1" "mining y -1"] -> w265
                  tunnel: ["mining angle 1" "mining angle -1"] -> w264
                  frame 1, Default {
                  }
                  frame -1 {
                  }
                }
                "mining x" <- w263
                "mining y" <- w265
                "mining angle" <- w264
                n94 = local write "x goal"(w263) -> ()
              }
              frame #1 {
                n95 = local read "state"() -> (w280:dbl)
                n96 = local write "stop motors"(0.0 ("stop motors")) -> ()
                n97 = Add(x=w280, y=1.0) -> (x+y=w282:dbl)
                n98 = local write "state"(w282) -> ()
              }
              frame #2 {
                n99 = local read "state"() -> (w285:dbl)
                n100 = Equal?(x=w285, y=1.0) -> (x = y?=w283:bool)
                n101 = call "Display Message to User"("Enable"=w283) -> ()  [unwired: 9 in, 2 out]
              }
            }
          }
          frame 1 {
            # "state 1=forward"
            n102 = while {
              stop <- w286 stop-if-true
              (unwired) FALSE
              n103 = flat-sequence {
                tunnel: [w295] -> w286
                frame #0 {
                  n104 = local write "stop motors"(1.0) -> ()
                }
                frame #1 {
                  n105 = while {
                    stop <- w290 stop-if-true
                    n106 = local read "x position 2"() -> (w288:dbl)
                    n107 = local read "x goal"() -> (w289:dbl)
                    n108 = Less Or Equal?(x=w288, y=w289) -> (x <= y?=w290:bool)
                  }
                }
                frame #2 {
                  n109 = local read "state"() -> (w291:dbl)
                  n110 = local write "stop motors"(0.0) -> ()
                  n111 = Add(x=w291, y=1.0) -> (x+y=w293:dbl)
                  n112 = local write "state"(w293) -> ()
                }
                frame #3 {
                  n113 = local read "state"() -> (w298:dbl)
                  n114 = Equal?(x=w298, y=2.0) -> (x = y?=w296:bool)
                  n115 = call "Display Message to User2"("Enable"=w296) -> ("OK"=w295:bool)  [unwired: 9 in, 1 out]
                }
              }
            }
          }
          frame 2 {
            # "state 2=dig"
            n116 = while {
              stop <- w299 stop-if-true
              n117 = flat-sequence {
                tunnel: [w310] -> w299
                frame #0 {
                  n118 = while {
                    stop <- w302 stop-if-true
                    n119 = shared-variable "RT myRIO Target - Overlord\\Mining_Variables_r0.lvlib\\Mining Complete"() -> (w301:bool)  [unwired: 1 in, 1 out]
                    n120 = shared-variable "RT myRIO Target - Overlord\\Mining_Variables_r0.lvlib\\Mine or Dump"(i16 1 ("Mine or Dump")) -> ()  [unwired: 1 in, 1 out]
                    n121 = Or(x=w301, y="digging complete?") -> (x .or. y?=w302:bool)
                  }
                }
                frame #1 {
                  n122 = local read "start x"() -> (w306:dbl)
                  n123 = local read "state"() -> (w308:dbl)
                  n124 = Add(x=w308, y=1.0) -> (x+y=w307:dbl)
                  n125 = Add(x=w306, y=1.0) -> (x+y=w305:dbl)
                  n126 = local write "x goal"(w305) -> ()
                  n127 = local write "state"(w307) -> ()
                }
                frame #2 {
                  n128 = local read "state"() -> (w313:dbl)
                  n129 = Equal?(x=w313, y=3.0) -> (x = y?=w311:bool)
                  n130 = call "Display Message to User8"("Enable"=w311) -> ("OK"=w310:bool)  [unwired: 9 in, 1 out]
                }
              }
            }
          }
          frame 3 {
            # "state 3=return"
            n131 = while {
              stop <- w314 stop-if-true
              (unwired) FALSE
              # "dialog for testing and move to next case"
              # "measurement and control"
              # "chill and make sure loc is good"
              # "house keeping variables"
              n132 = flat-sequence {
                tunnel: [w332] -> w314
                frame #0 {
                  n133 = local read "start x"() -> (w317:dbl)
                  n134 = local read "x goal"() -> (w315:dbl)
                  n135 = local read "right setpoint"() -> (w318:dbl)
                  n136 = local read "left setpoint"() -> (w319:dbl)
                  n137 = local write "stop motors"(1.0) -> ()
                  n138 = Subtract(x=w317, y=w315) -> (x-y=w316:dbl)
                  n139 = local write "right setpoint"(w319) -> ()
                  n140 = local write "left setpoint"(w318) -> ()
                  n141 = local write "x goal"(w316) -> ()
                }
                frame #1 {
                  n142 = while {
                    stop <- w324 stop-if-true
                    n143 = local read "x position 2"() -> (w321:dbl)
                    n144 = call "Elapsed Time9"() -> ("Time has Elapsed"=w323:bool)  [unwired: 12 in, 7 out]
                    n145 = local read "x goal"() -> (w322:dbl)
                    n146 = case shown="True" w323 {
                      frame False {
                      }
                      frame True {
                        n147 = flat-sequence {
                          frame #0 {
                            n148 = local write "stop motors"(0.0) -> ()
                          }
                          frame #1 {
                            n149 = Wait (ms)(milliseconds to wait=u32 1000) -> ()  [unwired: 1 out]
                          }
                          frame #2 {
                            n150 = local write "stop motors"(1.0) -> ()
                          }
                        }
                      }
                    }
                    n151 = Greater Or Equal?(x=w321, y=w322) -> (x >= y?=w324:bool)
                  }
                }
                frame #2 {
                  n152 = local read "state"() -> (w329:dbl)
                  n153 = local write "stop motors"(0.0) -> ()
                  n154 = Add(x=w329, y=1.0) -> (x+y=w331:dbl)
                  n155 = local write "state"(w331) -> ()
                }
                frame #3 {
                  n156 = local read "state"() -> (w335:dbl)
                  n157 = Equal?(x=w335, y=4.0) -> (x = y?=w333:bool)
                  n158 = call "Display Message to User5"("Enable"=w333) -> ("OK"=w332:bool)  [unwired: 9 in, 1 out]
                }
              }
            }
          }
          frame 4 {
            # "state 4=dump"
            n159 = flat-sequence {
              tunnel: [w345] -> w336
              frame #0 {
                n160 = while {
                  stop <- w339 stop-if-true
                  n161 = shared-variable "RT myRIO Target - Overlord\\Mining_Variables_r0.lvlib\\Dumping Complete"() -> (w338:bool)  [unwired: 1 in, 1 out]
                  n162 = shared-variable "RT myRIO Target - Overlord\\Mining_Variables_r0.lvlib\\Mine or Dump"(i16 -1 ("Mine or Dump")) -> ()  [unwired: 1 in, 1 out]
                  n163 = Or(x=w338, y="dumping complete") -> (x .or. y?=w339:bool)
                }
              }
              frame #1 {
                n164 = local read "mining location"() -> (w343:dbl)
                n165 = local write "state"(0.0) -> ()
                n166 = Multiply(x=w343, y=-1.0) -> (x*y=w341:dbl)
                n167 = local write "mining location"(w341) -> ()
              }
              frame #2 {
                n168 = local read "state"() -> (w348:dbl)
                n169 = Equal?(x=w348, y=0.0) -> (x = y?=w346:bool)
                n170 = call "Display Message to User9"("Enable"=w346) -> ("OK"=w345:bool)  [unwired: 9 in, 1 out]
              }
            }
          }
        }
      }
      n171 = while {
        tunnel: w202 -> [w486]
        tunnel: [w487] -> _
        tunnel: [w475] -> _
        shift-right: [w474] -> _
        shift-left: _ -> [w482]
        shift-right: ["pid reset right"] -> _
        shift-left: _ -> [w468]
        tunnel: w200 -> [w475]
        tunnel: w199 -> [w477]
        tunnel: w198 -> [w476]
        stop <- "pid reset right" stop-if-true
        # "******"
        n172 = local read "scale"() -> (w461:dbl)
        n173 = Greater?(x=w461, y=0.0) -> (0:w459:bool)
        n174 = case shown="True" w459 {
          tunnel: [w488 w489] -> w458
          frame False {
            n175 = local read "left setpoint"() -> (w488:dbl)
          }
          frame True {
            n176 = local read "right setpoint"() -> (w489:dbl)
          }
        }
        n177 = call "Elapsed Time"("Reset"=w468) -> ("Elapsed Time (s)"=w467:dbl, "Time has Elapsed"=w465:bool)  [unwired: 11 in, 6 out]
        "Elapsed Time (s) Right" <- w467
        n178 = local read "big red button"() -> (w454:i16)
        n179 = local read "encoder stop switch"() -> (w471:dbl)
        n180 = Not(x=w465) -> (.not. x?=w481:bool)
        ".not. x? 2" <- w481
        n181 = Greater Or Equal?(x=w467, y=4.0) -> (x >= y?=w464:bool)
        n182 = Multiply(x=w454, y=w458) -> (x*y=w455:dbl)
        n183 = case shown="False" w464 {
          tunnel: [1.0 1.0] -> w469
          frame False {
          }
          frame True {
          }
        }
        n184 = Multiply(x=w461, y=w455) -> (x*y=w473:dbl)
        n185 = local read "stop motors"() -> (w462:dbl)
        n186 = Multiply(x=w473, y=w471) -> (x*y=w472:dbl)
        n187 = Add(x=0.5, y=w473) -> (x+y=→"desired pwm right":dbl)
        n188 = Multiply(x=w462, y=w472) -> (x*y=w463:dbl)
        n189 = Multiply(x=w463, y=w469) -> (x*y=w470:dbl)
        n190 = call-poly <vilib>:"PID.vi"("reinitialize? (F)"=w481, "output range"="output range right", "PID gains"="PID gains right", "process variable"=w482, "setpoint"=w470) -> ("dt out (s)"=→"dt out (s) right":dbl, "output"=w474:dbl)  [unwired: 5 in]
        n191 = Add(x=0.5, y=w474) -> (x+y=w456:dbl)
        "right wheels actual pwm" <- w456
        "right pwm" <- w456
        n192 = call <vilib>:"Set Duty Cycle and Frequency.vi"("Frequency [Hz]"=w475, "Duty Cycle"=w456, "PWM Ref In"=w477) -> ()  [unwired: 6 in, 2 out]
        n193 = call <vilib>:"Set Duty Cycle and Frequency.vi"("Frequency [Hz]"=w475, "Duty Cycle"=w456, "PWM Ref In"=w476) -> ()  [unwired: 6 in, 2 out]
        n194 = call <vilib>:"Set Duty Cycle and Frequency.vi"("Frequency [Hz]"=w475, "Duty Cycle"=w456, "PWM Ref In"=w486) -> ("PWM Ref Out"=w487:T7)  [unwired: 6 in, 1 out]
        "PID feedback Right" <- w482
      }
      n195 = while {
        stop <- FALSE stop-if-true
        # "(current-start)/(goal-start)"
        n196 = local read "mining location"() -> (w216:dbl)
        n197 = case shown="-1, Default" w216 {
          frame 1 {
            "right setpoint" <- 0.05
            "left setpoint" <- 0.05
          }
          frame -1, Default {
            n198 = local write "right setpoint"(0.05) -> ()
            n199 = local write "left setpoint"(0.05) -> ()
          }
          frame 0 {
            w227 = 0.06 ("left setpoint")
            n200 = local write "right setpoint"(w227) -> ()
            n201 = local write "left setpoint"(w227) -> ()
          }
        }
        n202 = Not(x="motor killswitch") -> (.not. x?=w220:bool)
        n203 = local read "Encoder Reset"() -> (w222:bool)
        n204 = case shown="False" w222 {
          tunnel: [w237 w238] -> w221
          frame False {
            w237 = 1.0
            n205 = local write "reset x y 2"(w237) -> ()
          }
          frame True {
            w238 = 0.0
            n206 = local write "reset x y 2"(w238) -> ()
            "reset x y 2" <- w238
          }
        }
        "encoder stop switch" <- w221
        n207 = Boolean To (0,1)(Boolean=w220) -> (0, 1=→"big red button":i16)
        n208 = local read "x position 2"() -> (w215:dbl)
        n209 = local read "start x"() -> (w211:dbl)
        n210 = Subtract(x="x goal", y=w211) -> (x-y=w210:dbl)
        n211 = Subtract(x=w215, y=w211) -> (x-y=w214:dbl)
        n212 = Subtract(x=w211, y="x goal") -> (x-y=w213:dbl)
        n213 = Sign(1:w210) -> (0:w206:dbl)
        "scale" <- w206
        n214 = Divide(x=w214, y=w213) -> (x/y=w207:dbl)
        "percent to goal" <- w207
        n215 = Greater?(x=w207, y=0.75) -> (0:w208:bool)
        n216 = case shown="True" w208 {
          tunnel: w206 -> [w228 w230]
          tunnel: w207 -> [_ w231]
          frame False {
            n217 = Multiply(x=1.0, y=w228) -> ()  [unwired: 1 out]
          }
          frame True {
            n218 = Greater?(x=w231, y=1.001) -> (0:w232:bool)
            n219 = case shown="True" w232 {
              tunnel: w230 -> [w235 _]
              frame False {
                n220 = Multiply(x=w235, y=1.0) -> ()  [unwired: 1 out]
              }
              frame True {
                "goal reached" <- TRUE
              }
            }
          }
        }
      }
      n221 = while {
        shift-right: [w402] -> _
        shift-left: _ -> [w440]
        shift-right: [w399] -> _
        shift-left: _ -> [w439]
        shift-right: [w401] -> _
        shift-left: _ -> [w414]
        shift-right: [w400] -> _
        shift-left: _ -> [w413]
        stop <- FALSE stop-if-true
        w435 = 28.0  # width wheel to wheel
        w436 = 4.0  # wheel radius
        n222 = local read "reset x y 2"() -> (w398:dbl)
        n223 = call "Wait3"("Count(mSec)"=u32 20) -> ("Tick Count(mSec)"=→"Tick Count(mSec) 2":u32)
        n224 = Multiply(x=w398, y=w413) -> (x*y=w404:dbl)
        n225 = Multiply(x=w398, y=w440) -> (x*y=w406:dbl)
        n226 = Multiply(x=w398, y=w439) -> (x*y=w403:dbl)
        n227 = Multiply(x=w398, y=w414) -> (x*y=w405:dbl)
        n228 = local read "ENC.A_b.CNTR"() -> (w447:i32)
        n229 = local read "ENC.A_c.CNTR"() -> (w446:i32)
        n230 = local read "ENC.B_a.CNTR"() -> (w445:i32)
        n231 = local read "ENC.B_b.CNTR"() -> (w444:i32)
        n232 = local read "ENC.A_a.CNTR"() -> (w448:i32)
        n233 = local read "ENC.B_c.CNTR"() -> (w443:i32)
        n234 = Compound Arithmetic op=ADD(w448, w447, w446) -> (w452:i32)
        n235 = Compound Arithmetic op=ADD(w445, w444, w443) -> (w451:i32)
        n236 = Divide(x=w452, y=2) -> (x/y=w441:dbl)
        "avg ENC.A" <- w441
        n237 = Divide(x=w451, y=3) -> (x/y=w438:dbl)
        "avg ENC.B" <- w438
        n238 = Subtract(x=w441, y=w406) -> (x-y=w429:dbl)
        n239 = Subtract(x=w438, y=w403) -> (x-y=w428:dbl)
        n240 = Add(x=w429, y=w428) -> (x+y=w433:dbl)
        n241 = Divide(x=w436, y=w435) -> (x/y=w431:dbl)
        n242 = Square(x=w429) -> (x^2=w426:dbl)
        n243 = Square(x=w428) -> (x^2=w427:dbl)
        n244 = Subtract(x=w429, y=w428) -> (x-y=w432:dbl)
        n245 = Divide(x=w436, y=2.0) -> (x/y=w434:dbl)
        n246 = Add(x=w426, y=w427) -> (x+y=w425:dbl)
        n247 = Multiply(x=w432, y=w431) -> (x*y=→"psi dot 2":dbl)
        n248 = Multiply(x=w433, y=w434) -> (x*y=w422:dbl)
        n249 = Inverse Tangent(1:w432) -> (0:w430:dbl)
        n250 = Cosine(x=w430) -> (cos(x)=w423:dbl)
        n251 = Sine(x=w430) -> (sin(x)=w424:dbl)
        n252 = local read "reset x y 2"() -> (w396:dbl)
        n253 = Square Root(x=w425) -> (sqrt(x)=w419:dbl)
        n254 = Multiply(x=w422, y=w423) -> (x*y=w420:dbl)
        "x dot 2" <- w420
        n255 = Multiply(x=w422, y=w424) -> (x*y=w421:dbl)
        "y dot 2" <- w421
        n256 = Multiply(x=w441, y=w396) -> (x*y=w402:dbl)
        n257 = Multiply(x=w438, y=w396) -> (x*y=w399:dbl)
        n258 = Multiply(x=w419, y=w396) -> (x*y=w397:dbl)
        "distance traveled 2" <- w397
        n259 = Multiply(x=w397, y=w420) -> (x*y=w418:dbl)
        "x traveled 2" <- w418
        n260 = Multiply(x=w397, y=w421) -> (x*y=w417:dbl)
        "y traveled 2" <- w417
        n261 = Add(x=w404, y=w418) -> (x+y=w416:dbl)
        n262 = Add(x=w405, y=w417) -> (x+y=w408:dbl)
        n263 = Multiply(x=w416, y=w396) -> (x*y=w400:dbl)
        n264 = Multiply(x=w396, y=w408) -> (x*y=w401:dbl)
        n265 = Divide(x=w416, y=9600.0) -> (x/y=w411:dbl)
        n266 = Divide(x=w408, y=9600.0) -> (x/y=w412:dbl)
        n267 = local read "start x"() -> (w409:dbl)
        n268 = local read "start y"() -> (w410:dbl)
        n269 = Add(x=w411, y=w409) -> (x+y=→"x position 2":dbl)
        n270 = Add(x=w412, y=w410) -> (x+y=→"y position 2":dbl)
      }
      n271 = call "Tick Count"() -> ("Tick Count(uSec)"=w205:u32)
      n272 = while {
        shift-right: [w533] -> _
        shift-left: _ -> [w532]
        shift-right: [w530] -> _
        shift-left: w205 -> [w529]
        tunnel: w203 -> [w540]
        stop <- FALSE stop-if-true
        n273 = xnode "Read/Write Control"("FPGA VI Reference In"=w540) -> ("ENC.A_a.CNTR"=w539:u32, "ENC.A_b.CNTR"=w538:u32, "ENC.A_c.CNTR"=w537:u32, "ENC.B_a.CNTR"=w536:u32, "ENC.B_b.CNTR"=w535:u32, "ENC.B_c.CNTR"=w534:u32)  [unwired: 1 in, 2 out]
        n274 = call "Wait"("Count(mSec)"=u32 20) -> ()  [unwired: 1 out]
        n275 = Build Array(w539, w538, w537, w536, w535, w534) -> (w533:u32[])
        n276 = Subtract(x=w533, y=w532) -> (x-y=w531:u32[])
        n277 = call "Tick Count2"() -> ("Tick Count(uSec)"=w530:u32)
        n278 = Index Array(array=w531) -> (element #1=w528:u32, element #2=w527:u32, element #3=w526:u32, element #4=w525:u32, element #5=w524:u32, element #6=w523:u32)  [unwired: 6 in]
        n279 = Subtract(x=w530, y=w529) -> (x-y=w522:u32)
        n280 = call "Encoder-Velocity_Conversion (SubVI).vi"("delta  Encoder Count"=w528, "dt (uSec)"=w522) -> ("Rotational Velocity (RPS)"=w518:dbl)  [unwired: 7 in, 2 out]
        "LR Rot Velocity (rot/s)" <- w518
        n281 = call "Encoder-Velocity_Conversion (SubVI).vi"("delta  Encoder Count"=w523, "dt (uSec)"=w522) -> ("Rotational Velocity (RPS)"=w520:dbl)  [unwired: 7 in, 2 out]
        "RF Linear Velocity (rot/s)" <- w520
        n282 = call "Encoder-Velocity_Conversion (SubVI).vi"("delta  Encoder Count"=w527, "dt (uSec)"=w522) -> ("Rotational Velocity (RPS)"=w517:dbl)  [unwired: 7 in, 2 out]
        "LM Rot Velocity (rot/s)" <- w517
        n283 = call "Encoder-Velocity_Conversion (SubVI).vi"("delta  Encoder Count"=w526, "dt (uSec)"=w522) -> ("Rotational Velocity (RPS)"=w516:dbl)  [unwired: 7 in, 2 out]
        "LF Rot Velocity (rot/s)" <- w516
        n284 = call "Encoder-Velocity_Conversion (SubVI).vi"("delta  Encoder Count"=w525, "dt (uSec)"=w522) -> ("Rotational Velocity (RPS)"=w515:dbl)  [unwired: 7 in, 2 out]
        "RR Rot Velocity (rot/s)" <- w515
        n285 = call "Encoder-Velocity_Conversion (SubVI).vi"("delta  Encoder Count"=w524, "dt (uSec)"=w522) -> ("Rotational Velocity (RPS)"=w519:dbl)  [unwired: 7 in, 2 out]
        "RM Linear Velocity (rot/s)" <- w519
        n286 = Bundle("Rotational Velocity (RPS)"=w518, "Rotational Velocity (RPS)"=w517, "Rotational Velocity (RPS)"=w516, "Rotational Velocity (RPS)"=w515, "Rotational Velocity (RPS)"=w519, "Rotational Velocity (RPS)"=w520) -> (→"Current Rot Velocity (rot/s)":T4)  [unwired: 1 in]
      }
    }
  }
